vi "generateWaveform.vi"(8 "error in (no error)":errorcluster, 11 "chirp in":refnum<class "ChirpWave.lvclass">) -> (0 "error out":errorcluster, 2 "Signal Out":dbl, 3 "chirp out":refnum<class "ChirpWave.lvclass">)   [LabVIEW 2015, in "ChirpWave.lvclass"]
uses:
  ChirpWave.lvclass
  ChirpWave.lvclass/ChirpWave.ctl
  <vilib>/ptbypt/NI_PtbyPt.lvlib
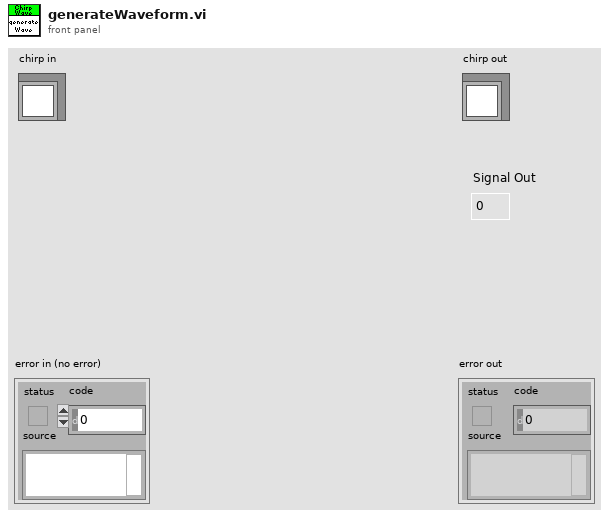
[diagram p1: front panel]
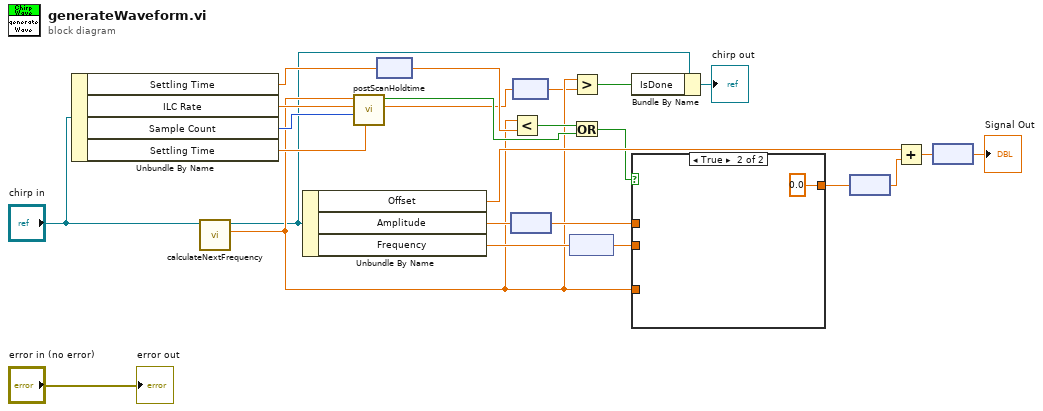
[diagram p0: block diagram]
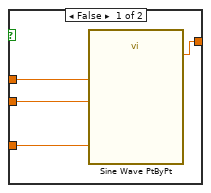
[diagram p2: hidden frame]
diagram:
  n1 = Unbundle By Name("chirp in") -> ("Settling Time"=w12:dbl[unit], "ILC Rate"=w13:dbl[unit], "Sample Count"=w11:u32, "Settling Time"=w10:dbl[unit])
  n2 = call "calculateNextFrequency.vi"("ChirpWave in"="chirp in") -> ("Delta Timestamp"=w6:dbl, "ChirpWave out"=w4:refnum<class "ChirpWave.lvclass">)  [unwired: 8 in, 1 out]
  n3 = Unbundle By Name(w4) -> ("Offset"=w22:dbl[unit], "Amplitude"=w24:dbl[unit], "Frequency"=w17:dbl[unit])
  n4 = call "postScanHoldtime.vi"("Settling Time"=w10, "Sample Count"=w11, "ILC Rate"=w13, "Delta"=w6) -> ("PostScan Hold time"=w2:dbl[unit], "Boolean"=w8:bool)  [unwired: 6 in]
  n5 = node(w12) -> (w14:dbl)
  n6 = node(w24) -> (w23:dbl)
  n7 = Less?(x=w6, y=w14) -> (x < y?=w9:bool)
  n8 = node(w2) -> (w1:dbl)
  n9 = node(w17) -> (w16:dbl)
  n10 = Greater?(x=w6, y=w1) -> (0:w5:bool)
  n11 = Or(x=w9, y=w8) -> (x .or. y?=w7:bool)
  n12 = Bundle By Name(cluster=w4, "IsDone"=w5) -> (→"chirp out":refnum<class "ChirpWave.lvclass">)
  n13 = case shown="True" w7 {
    tunnel: w23 -> [w29 _]
    tunnel: w16 -> [w26 _]
    tunnel: w6 -> [w28 _]
    tunnel: [w27 0.0 ("sine wave")] -> w21
    frame False {
      n14 = call <vilib>:"Sine Wave PtByPt.vi"("time"=w28, "frequency"=w26, "amplitude"=w29) -> ("sine wave"=w27:dbl)  [unwired: 1 in]
    }
    frame True {
    }
  }
  n15 = node(w21) -> (w20:dbl[unit])
  n16 = Add(x=w22, y=w20) -> (x+y=w19:dbl[unit])
  n17 = node(w19) -> (→"Signal Out":dbl)
  "error out" <- "error in (no error)"
